vi "Solve_Sub.vi"(4 "Entries":i32, 6 "Items":T1[](array[typedef]), 9 "Start":T1, 10 "End":T1, 11 "Width/Height":i32) -> (1 "map":T2[][](array[typedef]), 2 "key not found?":bool, 3 "Cost":u64)   [LabVIEW 2023, in "2024_18.lvclass"]
uses:
  2024_18.lvclass
  Tile18.ctl
  Common/AOC_XY(I32).ctl
  Common/AOC_Direction.ctl
  2024_18.lvclass/2024_18.ctl
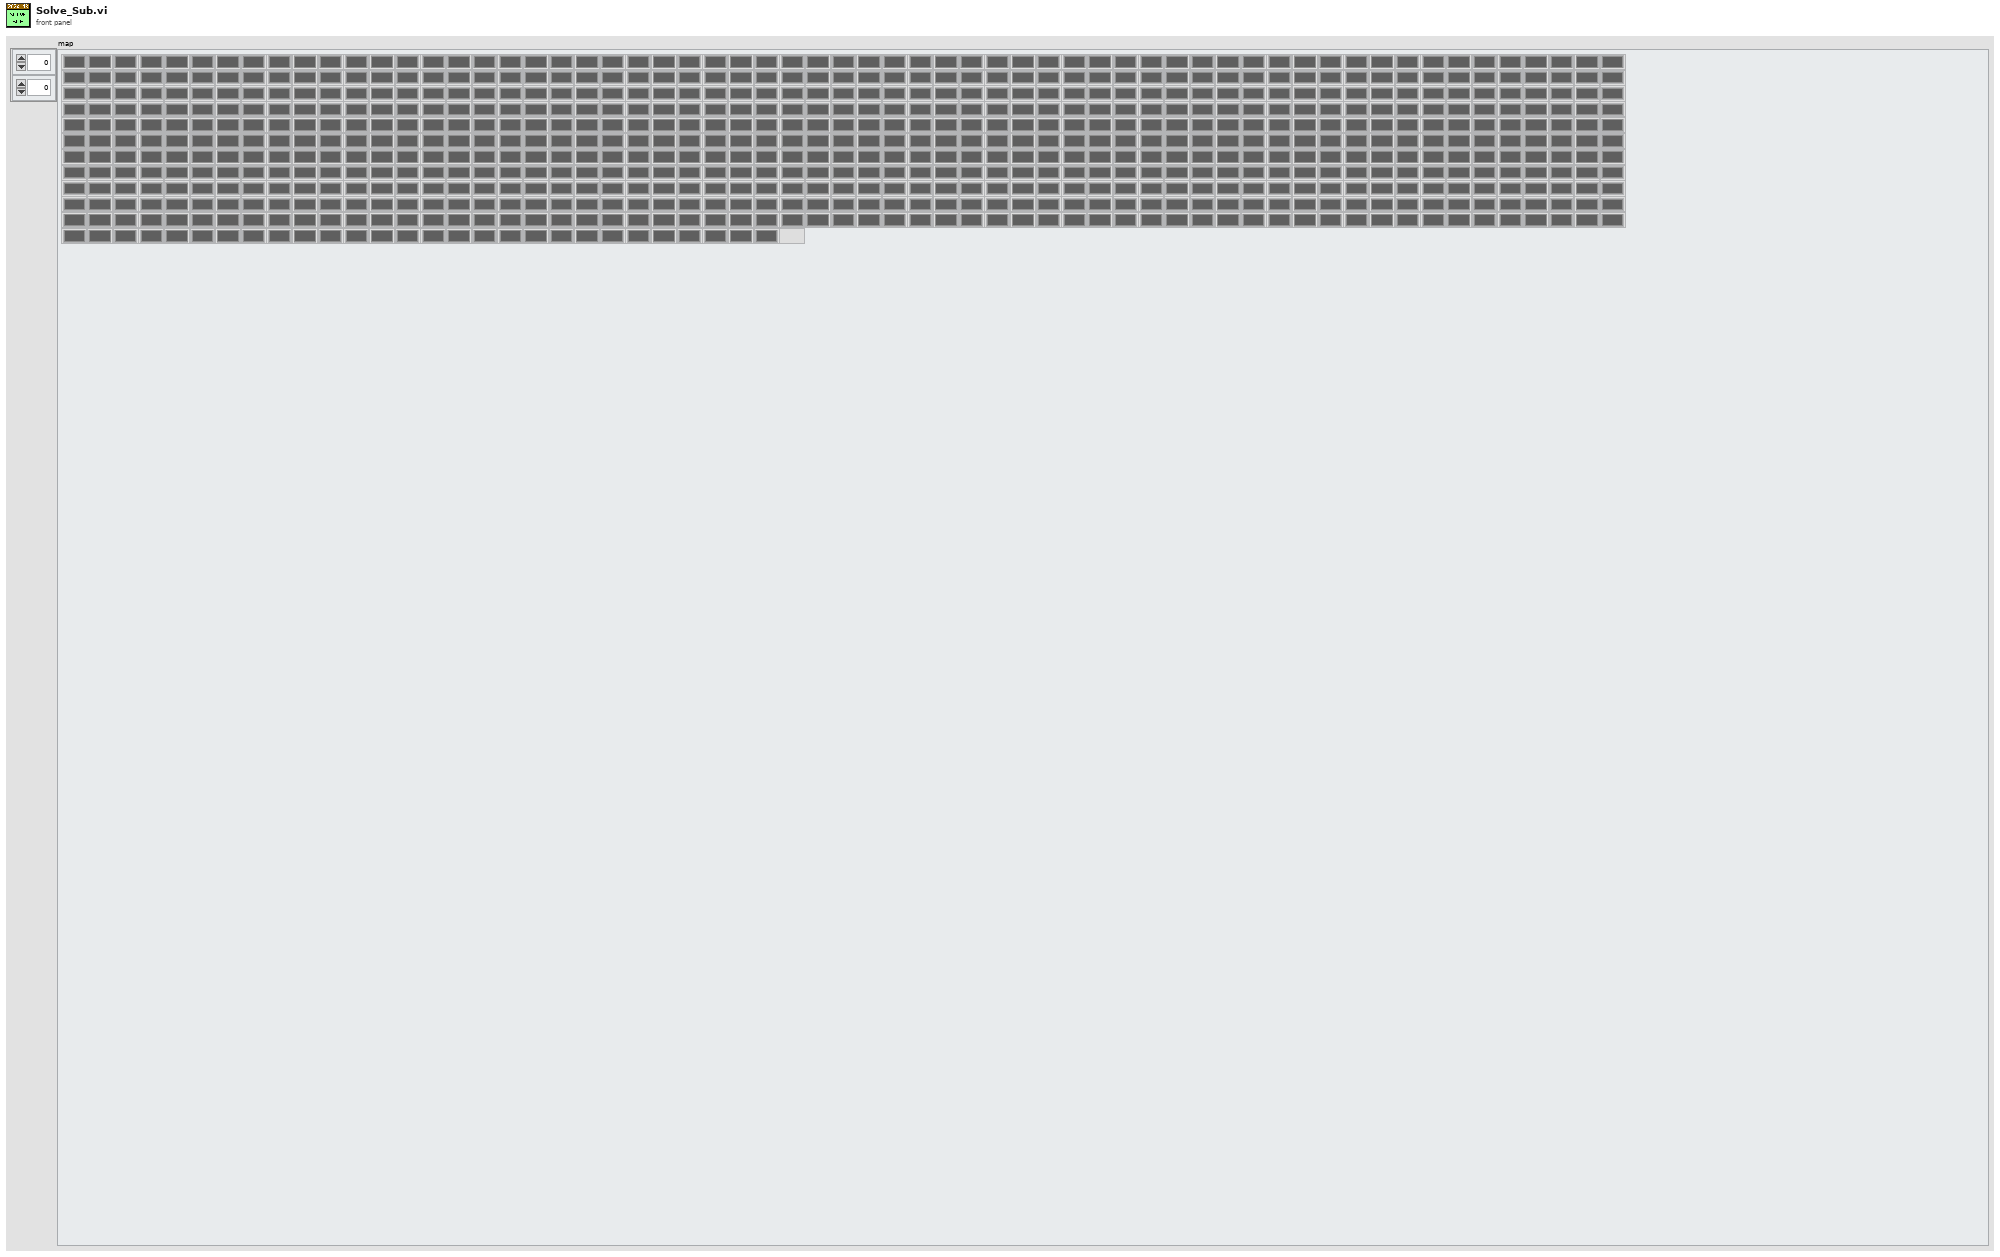
[diagram p1: front panel]
types:
  T1 = typedef "AOC_XY(I32).ctl" = cluster{"X":i32, "Y":i32}
  T2 = typedef "2024_18.lvclass/Tile18.ctl" = cluster{"Cost":i32, "BGColor":u32}
  T3 = typedef "AOC_Direction.ctl" = enum16{"Up", "Right", "Down", "Left"}
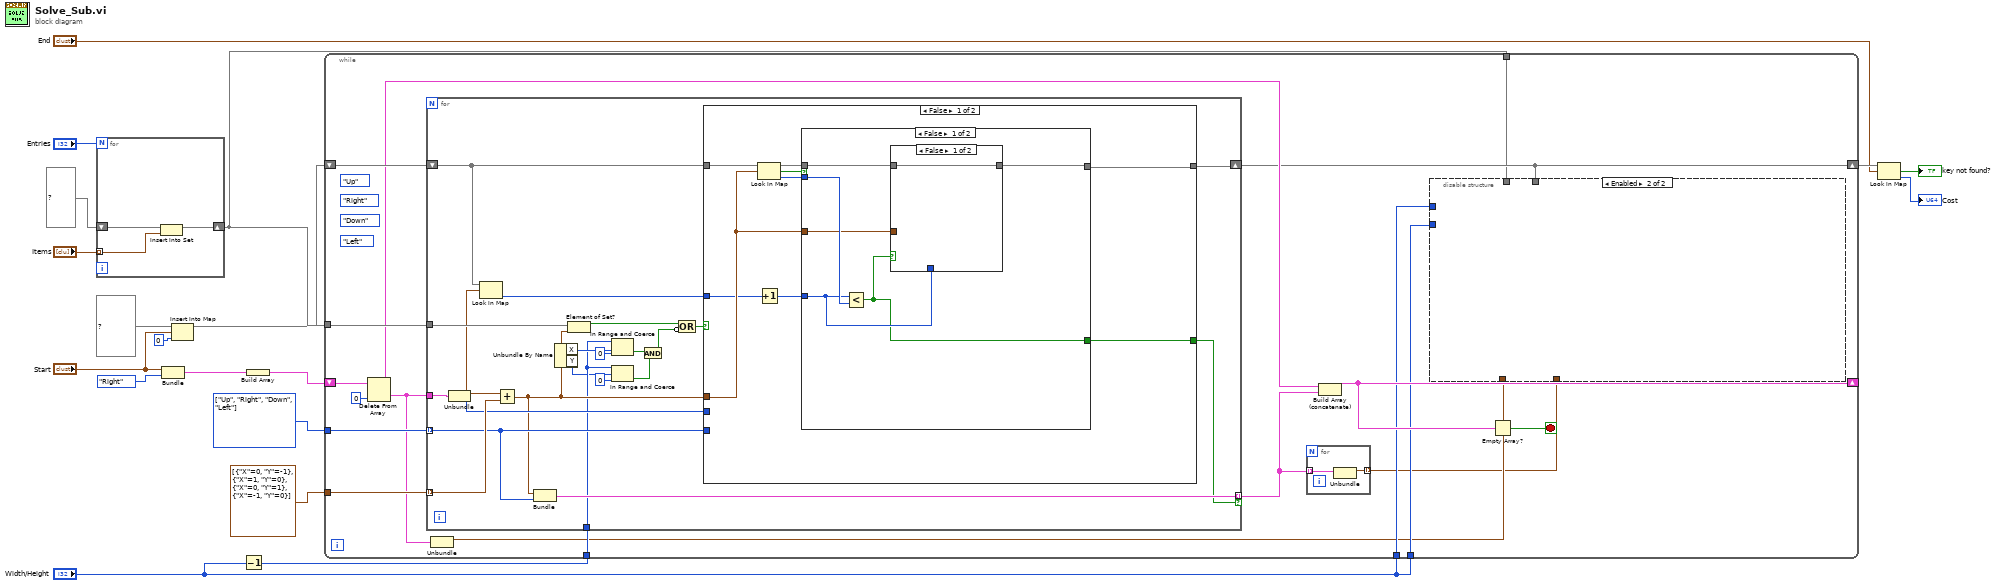
[diagram p0: block diagram]
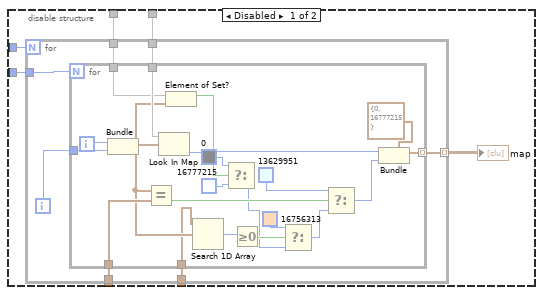
[diagram p2: hidden frame]
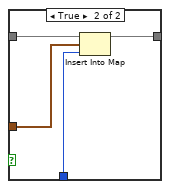
[diagram p3: hidden frame]
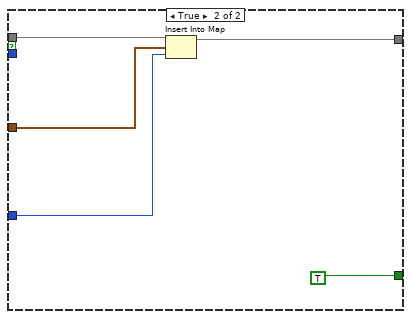
[diagram p4: hidden frame]
diagram:
  w4 = T3[] [enum."Up", enum."Right", enum."Down", enum."Left"] items=["Up", "Right", "Down", "Left"]
  n1 = for {
    N: "Entries" -> [_]
    tunnel: "Items" -> [w21] mode=indexing
    shift-right: [w20] -> w16
    shift-left: set{T1} {} ("set") -> [w22]
    n2 = Insert Into Set(10:w21, 11:w22) -> (3:w20:set{T1})  [unwired: 1 out]
  }
  n3 = Bundle("Start"="Start", AOC_Direction."Right") -> (w8:cluster{"Start":T1, T3})  [unwired: 1 in]
  n4 = Insert Into Map(map in=map{T1, u64} {} ("Cost"), key="Start", value=u64 0) -> (map out=w3:map{T1, u64})  [unwired: 2 out]
  n5 = Decrement(x="Width/Height") -> (x-1=w17:i32)
  n6 = Build Array(w8) -> (w2:cluster{"Start":T1, T3}[])
  n7 = while {
    shift-right: [w33] -> _
    shift-left: w2 -> [w40]
    shift-right: [w30] -> w10
    shift-left: w3 -> [w36]
    tunnel: w4 -> [w39]
    tunnel: cluster{"X":i32, "Y":i32}[] [{"X"=0, "Y"=-1}, {"X"=1, "Y"=0}, {"X"=0, "Y"=1}, {"X"=-1, "Y"=0}] ("Array") -> [w38]
    tunnel: w16 -> [w37]
    tunnel: "Width/Height" -> [w32]
    tunnel: "Width/Height" -> [w31]
    tunnel: w16 -> [w28]
    tunnel: w17 -> [w27]
    stop <- w29 stop-if-true
    (unwired) AOC_Direction."Left" ("Enum")
    (unwired) AOC_Direction."Down" ("Enum")
    (unwired) AOC_Direction."Right" ("Enum")
    (unwired) AOC_Direction."Up" ("Enum")
    n8 = Delete From Array(array=w40, index=0) -> (deleted portion=w26:cluster{"Start":T1, T3}, array with subset deleted=w35:cluster{"Start":T1, T3}[])  [unwired: 1 in]
    n9 = for {
      tunnel: w26 -> [w97]
      tunnel: w39 -> [w89] mode=indexing
      tunnel: w38 -> [w99] mode=indexing
      tunnel: w37 -> [w98]
      shift-right: [w96] -> w30
      shift-left: w36 -> [w92]
      tunnel: [w93] -> w24 mode=indexing if=w88
      tunnel: w27 -> [w83]
      n10 = Unbundle(w97) -> ("Start"=w91:T1, w94:T3)
      n11 = Look In Map(map=w92, key=w91) -> (value=w90:u64)  [unwired: 1 in, 1 out]
      n12 = Add(x=w91, y=w99) -> (x+y=w87:T1)
      n13 = Bundle("Start"=w87, "Enum"=w89) -> (w93:cluster{"Start":T1, "Enum":T3})  [unwired: 1 in]
      n14 = Unbundle By Name(w87) -> ("X"=w86:i32, "Y"=w82:i32)
      n15 = Element of Set?(10:w87, 11:w98) -> (3:w95:bool)
      n16 = In Range and Coerce(upper limit=w83, x=w86, lower limit=0) -> (In Range?=w81:bool)  [unwired: 1 out]
      n17 = In Range and Coerce(upper limit=w83, x=w82, lower limit=0) -> (In Range?=w80:bool)  [unwired: 1 out]
      n18 = And(x=w81, y=w80) -> (x .and. y?=w78:bool)
      n19 = Compound Arithmetic op=OR(w95, invert w78) -> (w79:bool)
      n20 = case shown="False" w79 {
        tunnel: w94 -> [_ _]
        tunnel: w89 -> [_ _]
        tunnel: w92 -> [w106 w124]
        tunnel: [w104 w124] -> w96
        tunnel: w87 -> [w105 _]
        tunnel: w90 -> [w102 _]
        tunnel: [w103 _] -> w88
        frame False {
          n21 = Look In Map(map=w106, key=w105) -> (key not found?=w107:bool, value=w100:u64)  [unwired: 1 in]
          n22 = Increment(x=w102) -> (x+1=w101:u64)
          n23 = case shown="False" w107 {
            tunnel: w106 -> [w112 w123]
            tunnel: w105 -> [w111 w122]
            tunnel: w101 -> [w110 w119]
            tunnel: [w109 w121] -> w104
            tunnel: [w108 TRUE] -> w103
            tunnel: w100 -> [w113 _]
            frame False {
              n24 = Less?(x=w110, y=w113) -> (x < y?=w108:bool)
              n25 = case shown="False" w108 {
                tunnel: w112 -> [w114 w118]
                tunnel: w111 -> [_ w117]
                tunnel: w110 -> [_ w116]
                tunnel: [w114 w115] -> w109
                frame False {
                }
                frame True {
                  n26 = Insert Into Map(map in=w118, key=w117, value=w116) -> (map out=w115:map{T1, u64})  [unwired: 2 out]
                }
              }
            }
            frame True {
              n27 = Insert Into Map(map in=w123, key=w122, value=w119) -> (map out=w121:map{T1, u64})  [unwired: 2 out]
            }
          }
        }
        frame True {
        }
      }
    }
    n28 = Unbundle(w26) -> ("Start"=w25:T1)  [unwired: 1 out]
    n29 = for {
      tunnel: w24 -> [w42] mode=indexing
      tunnel: [w41] -> w23 mode=indexing
      n30 = Unbundle(w42) -> ("Start"=w41:T1)  [unwired: 1 out]
    }
    n31 = Build Array (concatenate)(w35, w24) -> (w33:cluster{"Start":T1, "Enum":T3}[])
    n32 = disable-structure shown="Enabled" {
      disable-tunnel: w32 -> [w49 _]
      disable-tunnel: w31 -> [w48 _]
      disable-tunnel: w30 -> [w47 _]
      disable-tunnel: w28 -> [w45 _]
      disable-tunnel: w25 -> [w44 _]
      disable-tunnel: w23 -> [w43 _]
      frame Disabled {
        n33 = for {
          N: w48 -> [_]
          tunnel: w49 -> [w56]
          tunnel: w47 -> [w54]
          tunnel: [w53] -> w46 mode=indexing
          tunnel: w45 -> [w52]
          tunnel: w44 -> [w51]
          tunnel: w43 -> [w50]
          i -> [w55]
          n34 = for {
            N: w56 -> [_]
            tunnel: w55 -> [w76]
            tunnel: w54 -> [w75]
            tunnel: [w71] -> w53 mode=indexing
            tunnel: w52 -> [w70]
            tunnel: w51 -> [w68]
            tunnel: w50 -> [w62]
            i -> [w77]
            n35 = Bundle(w77, w76) -> (w63:cluster{i32, i32})  [unwired: 1 in]
            n36 = Equal?(x=w63, y=w68) -> (x = y?=w66:bool)
            n37 = Look In Map(map=w75, key=w63) -> (value=w73:u64)  [unwired: 1 in, 1 out]
            n38 = Element of Set?(10:w63, 11:w70) -> (3:w69:bool)
            n39 = Search 1D Array(1D array=w62, element=w63) -> (index of element=w61:i32)  [unwired: 1 in]
            n40 = Select(t=u32 0 ("BGColor"), s=w69, f=u32 16777215 ("BGColor")) -> (s? t:f=w58:u32)
            n41 = Greater Or Equal To 0?(x=w61) -> (x >= 0?=w60:bool)
            n42 = Select(t=u32 16756313 ("BGColor"), s=w60, f=w58) -> (s? t:f=w57:u32)
            n43 = Select(t=u32 13629951 ("BGColor"), s=w66, f=w57) -> (s? t:f=w64:u32)
            n44 = Bundle(cluster=T2 {"Cost"=0, "BGColor"=16777215} ("Cluster"), "Cost"=w73, "BGColor"=w64) -> (w71:T2)
          }
        }
        "map" <- w46
      }
      frame Enabled {
      }
    }
    n45 = Empty Array?(array=w33) -> (empty?=w29:bool)
  }
  n46 = Look In Map(map=w10, key="End") -> (key not found?=→"key not found?":bool, value=→"Cost":u64)  [unwired: 1 in]
